vi "FPGA Test.vi"() -> ()   [LabVIEW 2014]
uses:
  <vilib>/rvi/Emulation/niFpgaGetClockAttributes.vi
  <vilib>/rvi/Emulation/niFpgaSctlEmulationGetInTimedLoop.vi
  <vilib>/rvi/Emulation/niFpgaEmulationReportErrorSimple.vi
  <vilib>/rvi/eio/common/nirviEmuTemplateMethod_errors.vi
  <vilib>/rvi/Emulation/niFpgaCriticalErrorInLSC.vi
  <vilib>/eio/EIONode/EIONode.xnode
panel:
  out "result":bool
  in  "stop":bool
  in  "Test":bool
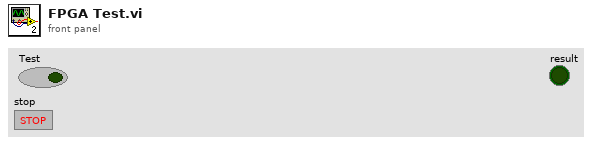
[diagram p1: front panel]
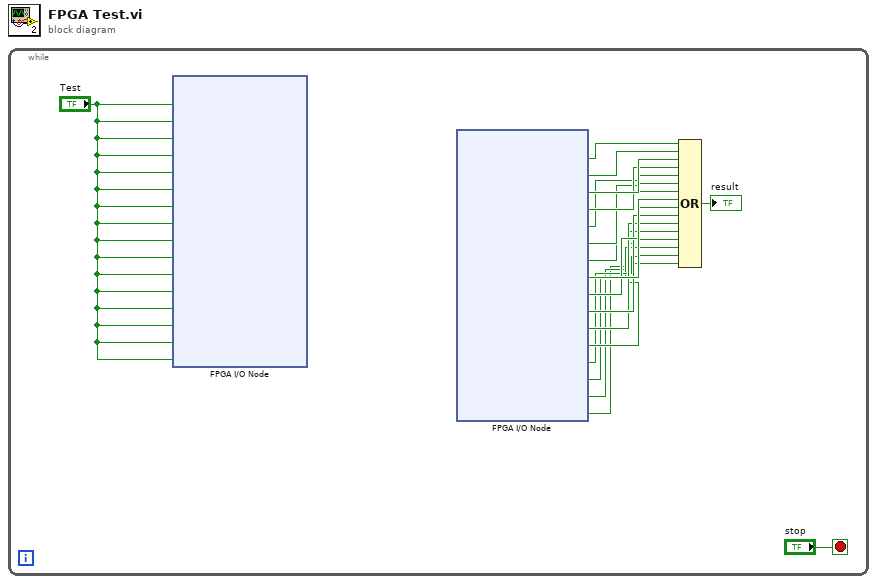
[diagram p0: block diagram]
diagram:
  n1 = while {
    stop <- "stop" stop-if-true
    n2 = xnode "FPGA I/O Node"("SSG Bkr Open"="Test", "SSG Bkr Close"="Test", "PV Bkr Open"="Test", "PV Bkr Close"="Test", "Gen West On/Off"="Test", "Gen East On/Off"="Test", "Mod2/DO6"="Test", "Mod2/DO7"="Test", "Mod2/DO8"="Test", "Mod2/DO9"="Test", "Mod2/DO10"="Test", "Mod2/DO11"="Test", "Mod2/DO12"="Test", "Mod2/DO13"="Test", "Mod2/DO14"="Test", "Mod2/DO15"="Test") -> ()  [unwired: 16 in, 16 out]
    n3 = xnode "FPGA I/O Node"() -> ("E-Stop Aux"=w17:bool, "PV Bkr Aux"=w16:bool, "SSG Bkr Aux"=w15:bool, "Mod2/DI3"=w14:bool, "Fire Alarm 1"=w13:bool, "Fire Alarm 2"=w12:bool, "Fire Fault"=w11:bool, "Gen Switch Off"=w10:bool, "Gen Switch On"=w9:bool, "Gen Switch Auto"=w8:bool, "Mod2/DI10"=w7:bool, "Mod2/DI11"=w6:bool, "Mod2/DI12"=w5:bool, "Mod2/DI13"=w4:bool, "Mod2/DI14"=w3:bool, "Mod2/DI15"=w2:bool)  [unwired: 16 in, 16 out]
    n4 = Compound Arithmetic op=OR(w17, w16, w15, w14, w13, w12, w11, w10, w9, w8, w7, w6, w5, w4, w3, w2) -> (→"result":bool)
  }
